vi "Entry.vi"(8 "error in (no error)":errorcluster, 11 "New State":refnum<class "Running Command.lvclass">) -> (0 "error out":errorcluster, 3 "State out":refnum<class "Running Command.lvclass">)   [LabVIEW 2014, in "Robot Actors.lvlib" / "Command Processor.lvlib" / "Running Command.lvclass"]
doc: "This is an abstract method. Override this method to define the behavior when you enter the state."
uses:
  Running Command.lvclass
  Command Processor Class/Command Processor States.ctl
  <vilib>/ActorFramework/Message Enqueuer/Message Enqueuer.lvclass/Message Enqueuer.ctl
  <vilib>/ActorFramework/Message Enqueuer/Enqueue.vi
  <vilib>/ActorFramework/Message Priority Queue/Priority Enqueue.vi
  Command/Command Messages/Start Command Msg/Start Command Msg.lvclass
  Command Processor Class/Command Processor.lvclass
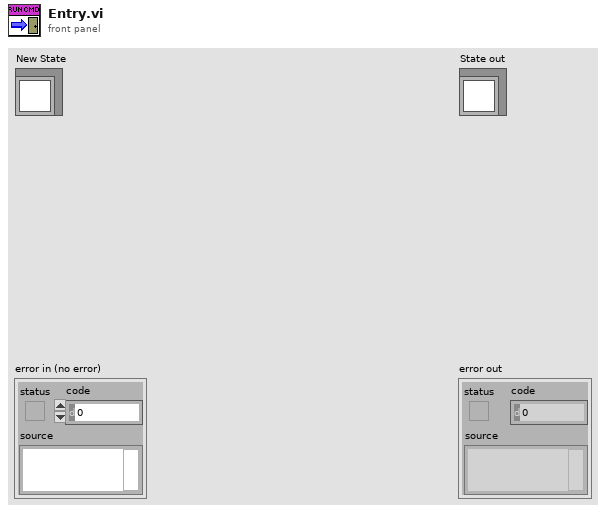
[diagram p1: front panel]
types:
  T1 = typedef "Robot Actors.lvlib/Command Processor.lvlib/Command Processor.lvclass/Command Processor States.ctl" = enum16{"Unknown", "No Command", "Running Command"}
  T2 = typedef "Robot Actors.lvlib/Command Processor.lvlib/Command Processor.lvclass/Command Processor Status.ctl" = cluster{"Next Command ID":dbl, "Current Command Status":T3, "Previous Command Status ":T3, "Command Processor State":T1, "Last Status Update":timestamp}
  T3 = typedef "Robot Actors.lvlib/Command.lvlib/Command.lvclass/Command Status.ctl" = cluster{"Command Name":string, "Command Start Time":timestamp, "Command End Time":timestamp, "Is Command Finished?":bool, "Command ID":dbl, "Command State":T4}
  T4 = typedef "Robot Actors.lvlib/Command.lvlib/Command.lvclass/Command States.ctl" = enum16{"Unknown", "Started", "Stopped", "Finished"}
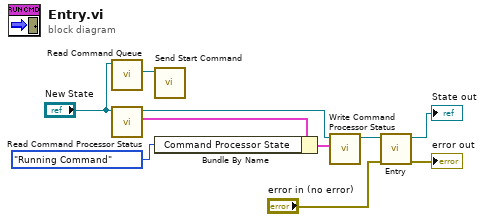
[diagram p0: block diagram]
diagram:
  n1 = call-dynamic "Read Command Queue.vi"("Command Processor in"="New State") -> ("Actor Framework:Message Enqueuer"=w7:refnum<class "Message Enqueuer.lvclass">)  [unwired: 8 in, 2 out]
  n2 = call-dynamic "Read Command Processor Status.vi"("Command Processor in"="New State") -> ("Command Processor Status"=w3:T2, "Command Processor out"=w6:refnum<class "Running Command.lvclass">)  [unwired: 8 in, 1 out]
  n3 = call "Send Start Command.vi"("Message Enqueuer"=w7) -> ()  [unwired: 9 in, 2 out]
  n4 = Bundle By Name(cluster=w3, "Command Processor State"=Command_Processor_States."Running Command") -> (w2:T2)
  n5 = call-dynamic "Write Command Processor Status.vi"("Command Processor Status"=w2, "Command Processor in"=w6) -> ("Command Processor out"=w4:refnum<class "Running Command.lvclass">)  [unwired: 8 in, 1 out]
  n6 = call-parent "Entry.vi"("error in (no error)"="error in (no error)", "New State"=w4) -> ("error out"=→"error out":errorcluster, "State out"=→"State out":refnum<class "Running Command.lvclass">)  [unwired: 8 in]
